vi "_DSF file plugins to data.vi"(8 "error in (no error)":errorcluster, 11 "configuration file cluster in":T1) -> (0 "error out":errorcluster, 2 "plugins":T9[](array[typedef]), 3 "configuration file cluster out":T1)   [LabVIEW 2017, in "DSF Configuration API v1.0.0.lvlib"]
uses:
  DSF Configuration API v1.0.0.lvlib
  Controls/dsf configuration file/1.0.0/dsf configuration.ctl
  Controls/dsf configuration file/1.0.0/version.ctl
  Controls/dsf configuration file/1.0.0/dsf plugin.ctl
  Controls/dsf configuration file/1.0.0/dsf timing.ctl
  Controls/dsf configuration file/1.0.0/dsf group.ctl
  Controls/dsf configuration file/1.0.0/dsf transfer.ctl
  Controls/dsf configuration file/1.0.0/dsf channel.ctl
  Controls/dsf configuration file/1.0.0/dsf settings.ctl
  Controls/dsf configuration data/1.0.0/dsf plugin.ctl
  Controls/dsf configuration data/1.0.0/dsf timing.ctl
  Controls/dsf configuration data/1.0.0/dsf group.ctl
  Controls/dsf configuration data/1.0.0/dsf transfer.ctl
  Controls/dsf configuration data/1.0.0/dsf channel.ctl
  Controls/dsf configuration data/1.0.0/dsf settings.ctl
  get item value by id/get setting value by id.vi
  Controls/dsf configuration data/1.0.0/dsf configuration data v1.0.0.lvlib
  Controls/dsf configuration file/1.0.0/dsf configuration file v1.0.0.lvlib
panel:
  # "dsf\nfile"
  # "dsf\nfile"
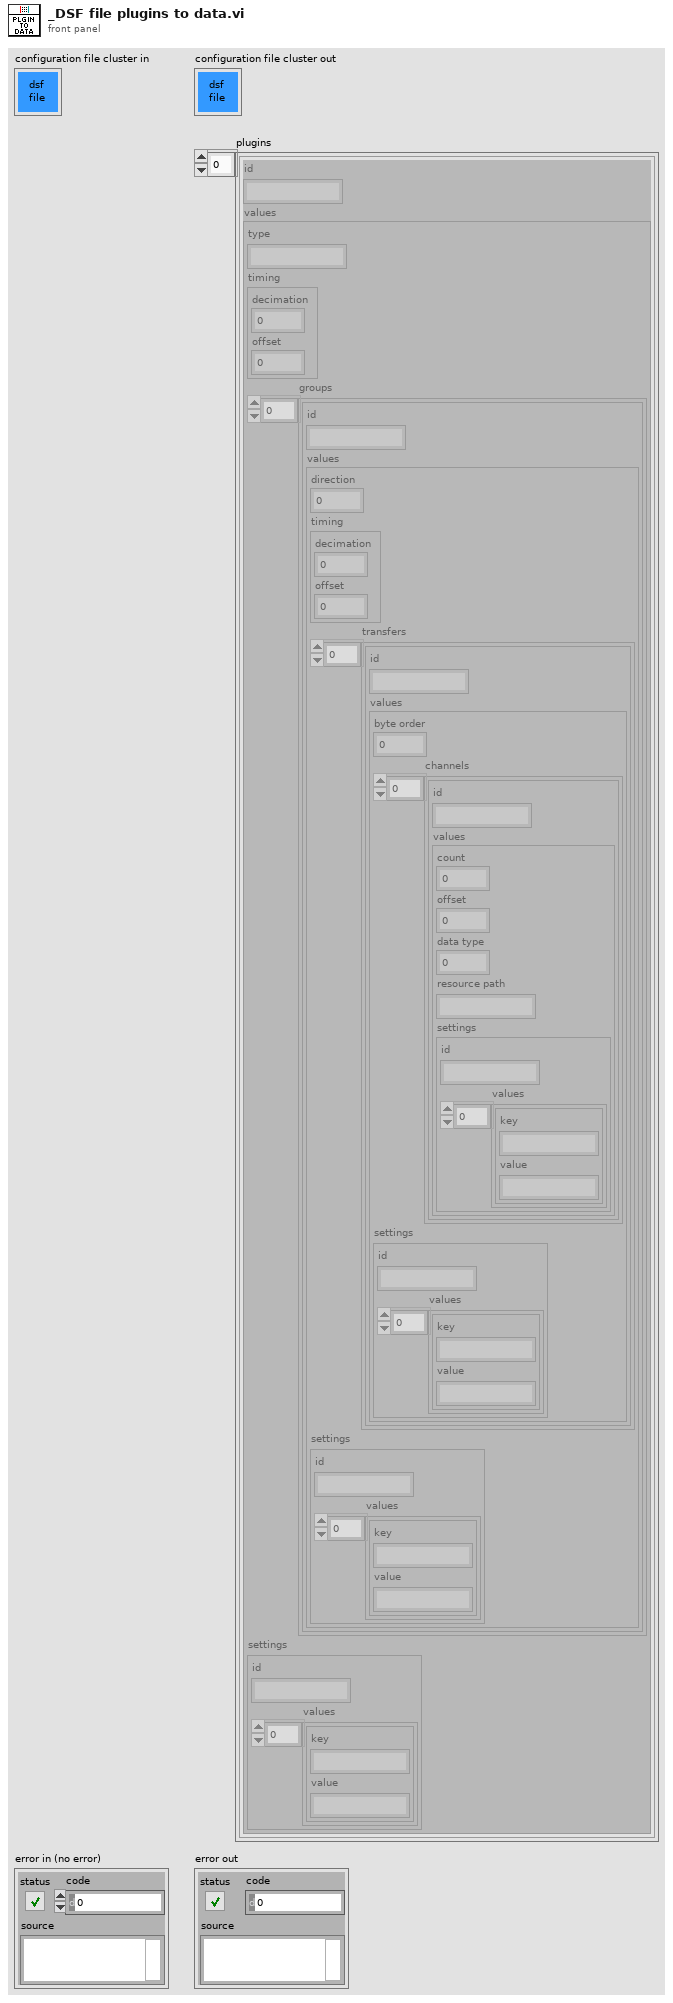
[diagram p1: front panel]
types:
  T1 = typedef "dsf configuration file v1.0.0.lvlib/dsf configuration.ctl" = cluster{"dsf":T2, "configuration":T2, "plugins":T3[], "groups":T5[], "transfers":T6[], "channels":T7[], "settings":T8[]}
  T2 = typedef "dsf configuration file v1.0.0.lvlib/version.ctl" = cluster{"major":u32, "minor":u32, "fix":u32, "build":string}
  T3 = typedef "dsf configuration file v1.0.0.lvlib/dsf plugin.ctl" = cluster{"id":string, "values":cluster{"type":string, "timing":T4, "group ids":string[], "settings id":string}}
  T4 = typedef "dsf configuration file v1.0.0.lvlib/dsf timing.ctl" = cluster{"decimation":i32, "offset":i32}
  T5 = typedef "dsf configuration file v1.0.0.lvlib/dsf group.ctl" = cluster{"id":string, "values":cluster{"direction":i32, "timing":T4, "transfer ids":string[], "settings id":string}}
  T6 = typedef "dsf configuration file v1.0.0.lvlib/dsf transfer.ctl" = cluster{"id":string, "values":cluster{"byte order":i32, "channel ids":string[], "settings id":string}}
  T7 = typedef "dsf configuration file v1.0.0.lvlib/dsf channel.ctl" = cluster{"id":string, "values":cluster{"count":i32, "offset":i32, "data type":i32, "resource path":string, "settings id":string}}
  T8 = typedef "dsf configuration file v1.0.0.lvlib/dsf settings.ctl" = cluster{"id":string, "values":cluster{"key":string, "value":string}[]}
  T9 = typedef "dsf configuration data v1.0.0.lvlib/dsf plugin.ctl" = cluster{"id":string, "values":cluster{"type":string, "timing":T10, "groups":T11[], "settings":T14}}
  T10 = typedef "dsf configuration data v1.0.0.lvlib/dsf timing.ctl" = cluster{"decimation":i32, "offset":i32}
  T11 = typedef "dsf configuration data v1.0.0.lvlib/dsf group.ctl" = cluster{"id":string, "values":cluster{"direction":i32, "timing":T10, "transfers":T12[], "settings":T14}}
  T12 = typedef "dsf configuration data v1.0.0.lvlib/dsf transfer.ctl" = cluster{"id":string, "values":cluster{"byte order":i32, "channels":T13[], "settings":T14}}
  T13 = typedef "dsf configuration data v1.0.0.lvlib/dsf channel.ctl" = cluster{"id":string, "values":cluster{"count":i32, "offset":i32, "data type":i32, "resource path":string, "settings":T14}}
  T14 = typedef "dsf configuration data v1.0.0.lvlib/dsf settings.ctl" = cluster{"id":string, "values":cluster{"key":string, "value":string}[]}
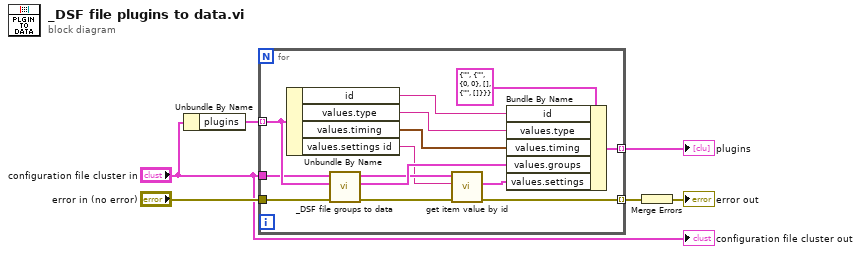
[diagram p0: block diagram]
diagram:
  n1 = Unbundle By Name("configuration file cluster in") -> ("plugins"=w3:T3[])
  n2 = for {
    tunnel: w3 -> [w14] mode=indexing
    tunnel: "configuration file cluster in" -> [w9]
    tunnel: [w15] -> w1 mode=indexing
    tunnel: "error in (no error)" -> [w13]
    tunnel: [w11] -> w5 mode=indexing
    n3 = Unbundle By Name(w14) -> ("id"=w19:string, "values.type"=w18:string, "values.timing"=w17:T4, "values.settings id"=w7:string)
    n4 = call "_DSF file groups to data.vi"("error in (no error)"=w13, "plugin"=w14, "configuration file cluster in"=w9) -> ("error out"=w12:errorcluster, "groups"=w10:T11[], "configuration file cluster out"=w8:T1)  [unwired: 6 in]
    n5 = call-poly "get item value by id.vi"("error in (no error)"=w12, "id"=w7, "configuration file cluster in"=w8) -> ("error out"=w11:errorcluster, "settings"=w16:T8)  [unwired: 5 in, 2 out]
    n6 = Bundle By Name(cluster=T9 {"id"="", "values"={"type"="", "timing"={"decimation"=0, "offset"=0}, "groups"=[], "settings"={"id"="", "values"=[]}}} ("plugin"), "id"=w19, "values.type"=w18, "values.timing"=w17, "values.groups"=w10, "values.settings"=w16) -> (w15:T9)
  }
  "plugins" <- w1
  n7 = Merge Errors(w5) -> (→"error out":errorcluster)
  "configuration file cluster out" <- "configuration file cluster in"
